vi "Create Graph Data.vi"(8 "error in (no error)":errorcluster, 9 "Signal":string, 10 "LogPath":path, 11 "Test Data":T1[](array[typedef])) -> (0 "error out":errorcluster, 1 "Idx":i32, 2 "Graph Data":dbl[][](array[numeric]), 3 "Test Data dup":T1[](array[typedef]), 5 "System Time":dbl[](array[numeric]))   [LabVIEW 2011]
uses:
  Controls/Test Column Data.ctl
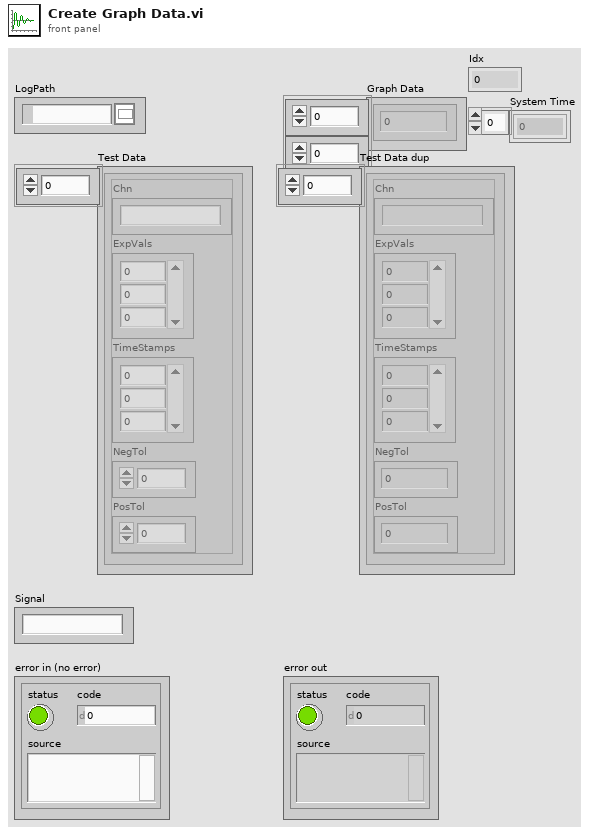
[diagram p1: front panel]
types:
  T1 = typedef "Test Column Data.ctl" = cluster{"Chn":string, "ExpVals":dbl[], "TimeStamps":i64[], "NegTol":dbl, "PosTol":dbl}
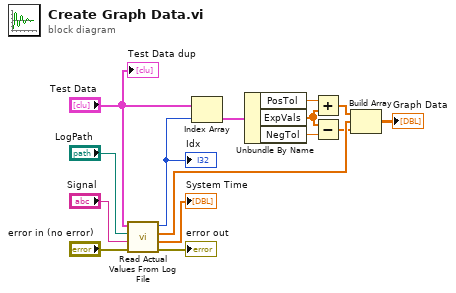
[diagram p0: block diagram]
diagram:
  n1 = call "Read Actual Values From Log File.vi"("Error In"="error in (no error)", "Signal"="Signal", "Log"="LogPath", "Test Data"="Test Data") -> ("Error Out"=→"error out":errorcluster, "System Time"=→"System Time":dbl[], "Actual Values"=w13:dbl[], "Idx"=w6:i32)  [unwired: 4 in]
  "Idx" <- w6
  n2 = Index Array(array="Test Data", index=w6) -> (element=w7:T1)
  n3 = Unbundle By Name(w7) -> ("PosTol"=w8:dbl, "ExpVals"=w9:dbl[], "NegTol"=w10:dbl)
  n4 = Add(x=w8, y=w9) -> (x+y=w12:dbl[])
  n5 = Subtract(x=w9, y=w10) -> (x-y=w11:dbl[])
  n6 = Build Array(w12, w13, w11) -> (→"Graph Data":dbl[][])
  "Test Data dup" <- "Test Data"
